vi "SETNCdll.vi"(8 "error in (no error)":errorcluster, 11 "ncomp":i32) -> (0 "error out":errorcluster, 3 "ncomp out":i32)   [LabVIEW 2021]
doc: "subroutine SETNC (ncomp)\n\n Allow the user to modify the value of ncomp (the number of components in\n a mixture) so that a subset of the full setup can be used.\n For example, a 5 component mixture could be set up, but nc could\n be set to 3 to calculate properties for just the first three components.\n This also allows a mixture to be setup with one or more pure fluids\n loaded after the components in the mixture. For example, R407C could\n be loaded by calling setup with R32.fld, R125.fld, R134a.fld, and R407C.ppf.\n The number of components would be set to 3, and PUREFLD would be called\n to access the properties from component 4, the pseudo-pure fluid equation.\n\nINPUTS:\nncomp--number of components in the mixture"
uses:
  REFPROP.dll
panel:
  # "REFPROP-SETNCdll.vi"
  # "void  SETNCdll(int32_t *ncomp);"
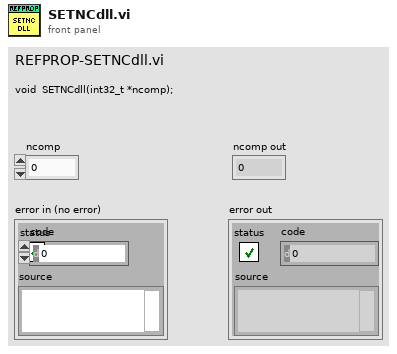
[diagram p1: front panel]
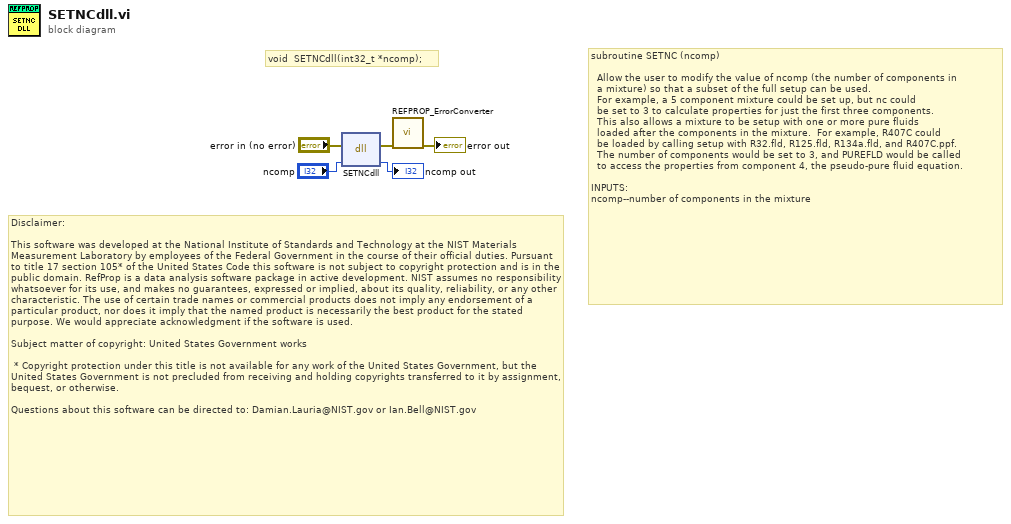
[diagram p0: block diagram]
diagram:
  # "Disclaimer:\n\nThis software was developed at the National Institute of Standards and Technology at the NIST Materials Measurement Laboratory by employees of the Federal Government in the course of their official duties. Pursuant to title 17 section 105* of the United States Code this software is not subject to copyright protection and is in the public domain. RefProp is a data analysis software package in active development. NIST assumes no responsibility whatsoever for its use, and makes no guarantees, expressed or implied, about its quality, reliability, or any other characteristic. The use of certain trade names or commercial products does not imply any endorsement of a particular product, nor does it imply that the named product is necessarily the best product for the stated purpose. We would appreciate acknowledgment if the software is used.\n \nSubject matter of copyright: United States Government works\n  \n * Copyright protection under this title is not available for any work of the United States Government, but the United States Government is not precluded from receiving and holding copyrights transferred to it by assignment, bequest, or otherwise.\n\nQuestions about this software can be directed to: Damian.Lauria@NIST.gov or Ian.Bell@NIST.gov"
  # "void  SETNCdll(int32_t *ncomp);"
  # "subroutine SETNC (ncomp)\n\n  Allow the user to modify the value of ncomp (the number of components in\n  a mixture) so that a subset of the full setup can be used.\n  For example, a 5 component mixture could be set up, but nc could\n  be set to 3 to calculate properties for just the first three components.\n  This also allows a mixture to be setup with one or more pure fluids\n  loaded after the components in the mixture.  For example, R407C could\n  be loaded by calling setup with R32.fld, R125.fld, R134a.fld, and R407C.ppf.\n  The number of components would be set to 3, and PUREFLD would be called\n  to access the properties from component 4, the pseudo-pure fluid equation.\n\nINPUTS:\nncomp--number of components in the mixture"
  n1 = dll-call lib="C:/Users/lauria/OneDrive - National Institute of Standards and Technology (NIST)/LabVIEW Projects/7 REFPROP/REFPROP-wrappers-master/REFPROP-wrappers-master/wrappers/Labview/REFPROP/REFPROP.*" fn="SETNCdll"(error in="error in (no error)", "ncomp"="ncomp") -> (error out=w3:errorcluster, "ncomp"=→"ncomp out":i32)  [unwired: 3 in, 1 out]
  n2 = call "REFPROP_ErrorConverter.vi"("error in (no error)"=w3) -> ("error out"=→"error out":errorcluster)  [unwired: 10 in]
